vi "Image-correlation.vi"(6 "Image index":i32, 8 "error in":errorcluster, 9 "Correct. params. ref. in":refnum<data-value>, 10 "Buffer element in":T1 {"Temperature characteristics"."Stand. dev. temperature" format="%#.1f"; "Temperature characteristics"."Min. temperature" format="%#.0f"; "Temperature characteristics"."Max. temperature" format="%#.0f"; "Temperature characteristics"."Average temperature" format="%#.0f"}) -> (0 "error IO":errorcluster, 1 "Correct. params. ref.":refnum<data-value>, 2 "Buffer element":T1 {"Temperature characteristics"."Stand. dev. temperature" format="%#.1f"; "Temperature characteristics"."Min. temperature" format="%#.0f"; "Temperature characteristics"."Max. temperature" format="%#.0f"; "Temperature characteristics"."Average temperature" format="%#.0f"})   [LabVIEW 2013, in "CameraVision.lvlib" / "CV-Main.lvclass"]
uses:
  CV-Main.lvclass
  Correction/CV-Correction.lvclass
  Buffers/Storage-buffer.ctl
  <vilib>/vision/Image Controls.llb/IMAQ Image.ctl
  Temperature/Temperature-characteristics.ctl
  Analysis/Characteristics-cluster.ctl
  Correction/CV-Correction.lvclass/CV-Correction.ctl
  Correction/Read X-shift.vi
  Correction/Read Y-shift.vi
  Correction/Read Cross-correlation algorithm.vi
  Correction/Read Cross-correlation decimation.vi
  Correction/Write Image shift.vi
  Correction/Read Correlation algorithm.vi
  Correction/Read 2nd image correlation.vi
  Correction/Read 2nd image mirror axis.vi
  <vilib>/vision/NI_Vision_Development_Module.lvlib
  Temperature/CV-Temperature.lvclass
  Analysis/CV-Analysis.lvclass
  Buffers/CV-Buffers.lvclass
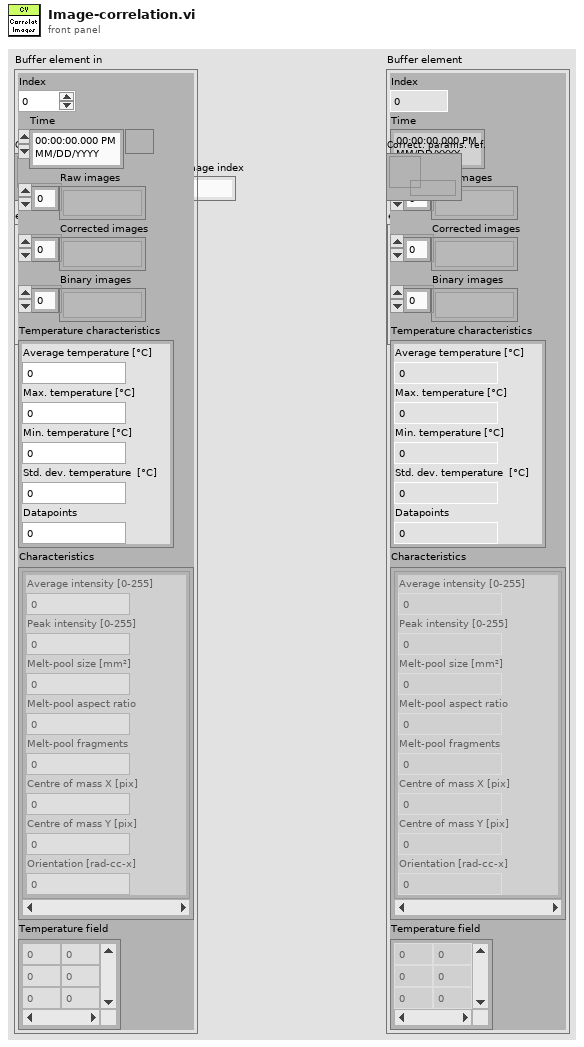
[diagram p1: front panel]
types:
  T1 = typedef "CameraVision.lvlib/CV-Buffers.lvclass/Storage-buffer.ctl" = cluster{"Index":i32, "Time":timestamp, "Raw images":T2[], "Corrected images":T2[], "Binary images":T2[], "Temperature characteristics":T3, "Characteristics":T4[], "Temperature field":dbl[][]}
  T2 = typedef "IMAQ Image.ctl" = refnum<image>
  T3 = typedef "CameraVision.lvlib/CV-Temperature.lvclass/Temperature-characteristics.ctl" = cluster{"Average temperature ":dbl, "Max. temperature":dbl, "Min. temperature":dbl, "Stand. dev. temperature":dbl, "Datapoints":dbl}
  T4 = typedef "CameraVision.lvlib/CV-Analysis.lvclass/Characteristics-cluster.ctl" = cluster{"Average intensity":dbl, "Peak intensity":dbl, "Melt-pool size":dbl, "Melt-pool aspect ratio":dbl, "Melt-pool fragments":dbl, "Centre of mass X":dbl, "Centre of mass Y":dbl, "Orientation":dbl}
  T5 = enum16{"Fixed shift", "Cross-correlation", "Cross-correlation (5steps)", "Melt-pool center"}
  T6 = cluster{"Accessors RO:X-shift":i32, "Accessors RO:Y-shift":i32}
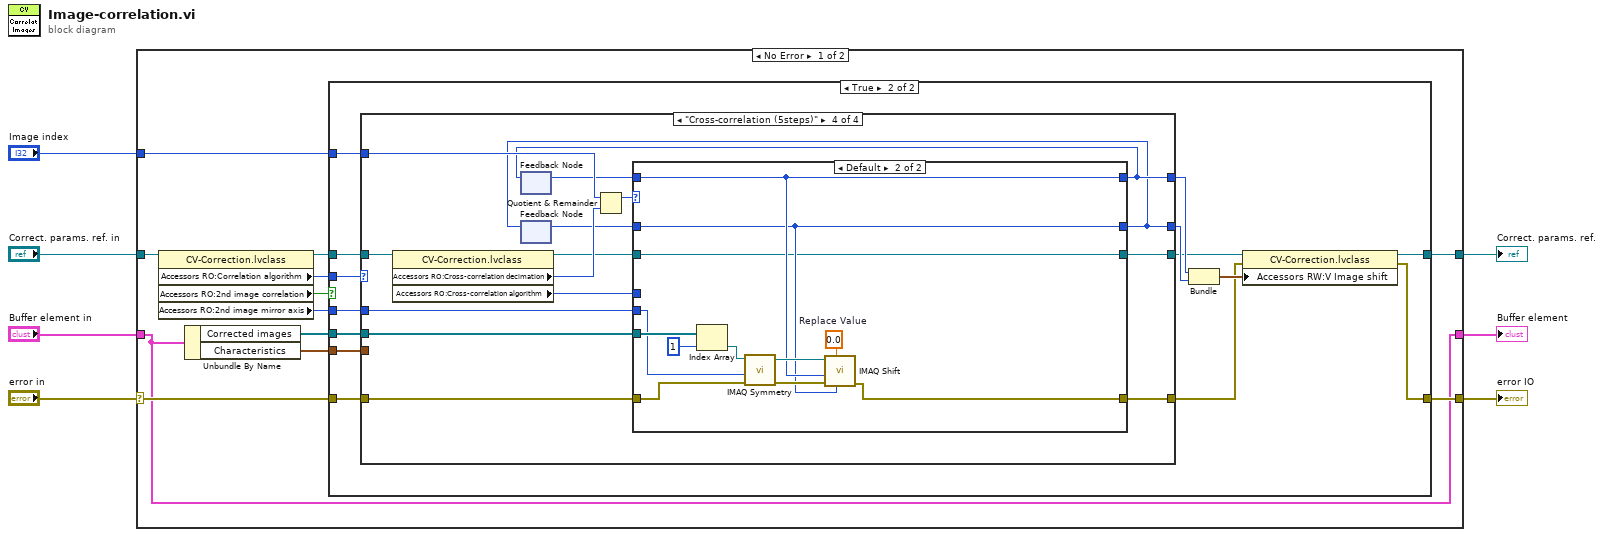
[diagram p0: block diagram]
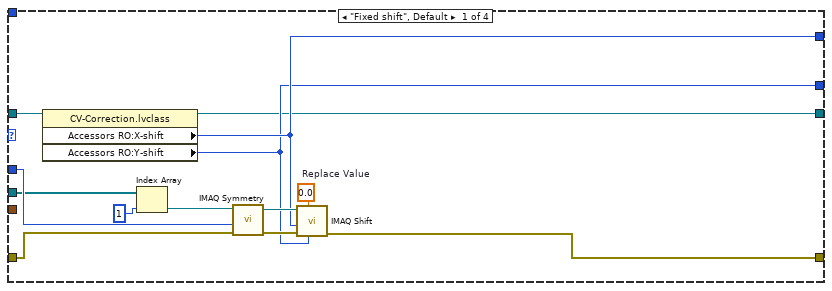
[diagram p3: hidden frame]
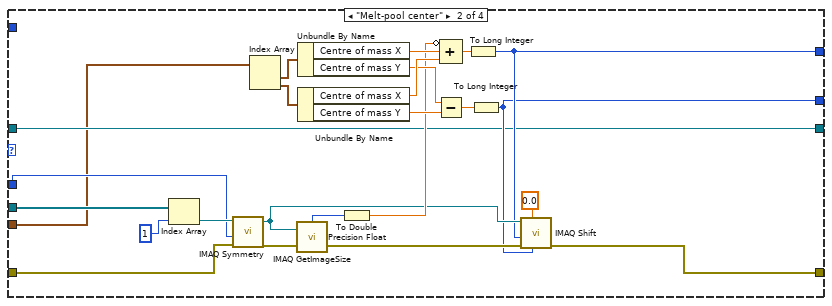
[diagram p4: hidden frame]
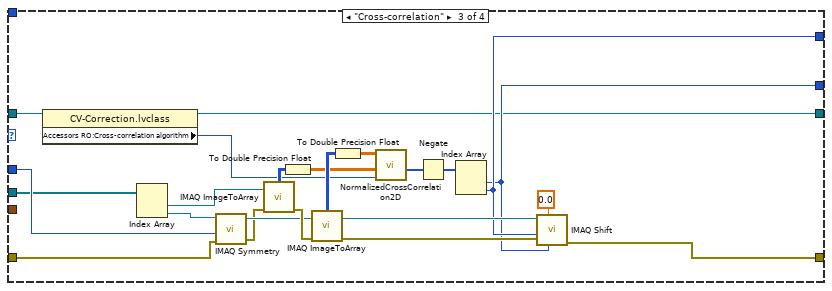
[diagram p5: hidden frame]
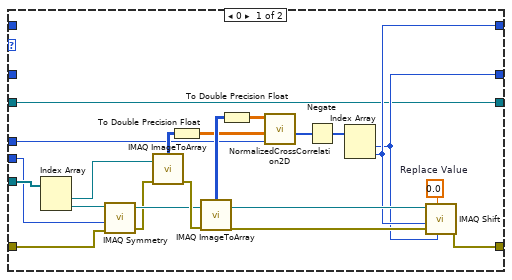
[diagram p6: hidden frame]
diagram:
  n1 = case shown="No Error" "error in" {
    selector: "error in" -> [w11 w145]
    tunnel: "Image index" -> [w19 _]
    tunnel: "Correct. params. ref. in" -> [w16 w144]
    tunnel: [w18 w145] -> w6
    tunnel: "Buffer element in" -> [w9 w143]
    tunnel: [w12 w144] -> w2
    tunnel: [w9 w143] -> w1
    frame No Error {
      n2 = property class="CV-Correction.lvclass"(reference=w16) -> (reference out=w17:refnum<data-value>, "Accessors RO:Correlation algorithm"=w15:T5, "Accessors RO:2nd image correlation"=w14:bool, "Accessors RO:2nd image mirror axis"=w13:u32)  [unwired: 1 in, 1 out]
      n3 = Unbundle By Name(w9) -> ("Corrected images"=w10:T2[], "Characteristics"=w8:T4[])
      n4 = case shown="True" w14 {
        tunnel: w19 -> [_ w35]
        tunnel: w15 -> [_ w34]
        tunnel: w17 -> [w21 w33]
        tunnel: [w20 w26] -> w18
        tunnel: w13 -> [_ w32]
        tunnel: [w21 w28] -> w12
        tunnel: w11 -> [w20 w24]
        tunnel: w10 -> [_ w23]
        tunnel: w8 -> [_ w22]
        frame False {
        }
        frame True {
          n5 = case shown="\"Cross-correlation (5steps)\"" w34 {
            tunnel: [w39 w53 w76 w107] -> w25
            tunnel: w33 -> [w42 w52 w81 w106]
            tunnel: w35 -> [_ _ _ w109]
            tunnel: w32 -> [w43 w57 w79 w102]
            tunnel: [w41 w55 w78 w101] -> w31
            tunnel: [w40 w54 w77 w99] -> w30
            tunnel: [w38 w52 w75 w97] -> w29
            tunnel: w24 -> [w36 w51 w74 w96]
            tunnel: w23 -> [w37 w50 w73 w95]
            tunnel: w22 -> [_ w49 _ _]
            frame "Fixed shift", Default {
              w48 = sgl 0.0  # Replace Value
              n6 = property class="CV-Correction.lvclass"(reference=w42) -> (reference out=w38:refnum<data-value>, "Accessors RO:X-shift"=w41:i32, "Accessors RO:Y-shift"=w40:i32)  [unwired: 1 in, 1 out]
              n7 = Index Array(array=w37, index=1) -> (element=w47:T2)
              n8 = call "IMAQ Symmetry"("error in (no error)"=w36, "Type of Symmetry"=w43, "Image Src"=w47) -> ("error out"=w44:errorcluster, "Image Dst Out"=w45:T2)  [unwired: 2 in]
              n9 = call "IMAQ Shift"("YOffset"=w40, "Replace Value"=w48, "error in (no error)"=w44, "XOffset"=w41, "Image Src"=w45) -> ("error out"=w39:errorcluster)  [unwired: 5 in, 1 out]
            }
            frame "Melt-pool center" {
              n10 = Index Array(array=w50, index=1) -> (element=w63:T2)
              n11 = call "IMAQ Symmetry"("error in (no error)"=w51, "Type of Symmetry"=w57, "Image Src"=w63) -> ("error out"=w61:errorcluster, "Image Dst Out"=w56:T2)  [unwired: 2 in]
              n12 = Index Array(array=w49) -> (element #1=w72:T4, element #2=w71:T4)  [unwired: 2 in]
              n13 = call "IMAQ GetImageSize"("Image"=w56, "error in (no error)"=w61) -> ("X Resolution"=w59:i32, "error out"=w60:errorcluster)  [unwired: 2 in, 1 out]
              n14 = Unbundle By Name(w72) -> ("Centre of mass X"=w70:dbl, "Centre of mass Y"=w67:dbl)
              n15 = Unbundle By Name(w71) -> ("Centre of mass X"=w69:dbl, "Centre of mass Y"=w68:dbl)
              n16 = To Double Precision Float(number=w59) -> (double precision float=w58:dbl)
              n17 = Subtract(x=w67, y=w68) -> (x-y=w65:dbl)
              n18 = Compound Arithmetic op=ADD(invert w58, w70, w69) -> (w66:dbl)
              n19 = To Long Integer(number=w66) -> (32bit integer=w55:i32)
              n20 = To Long Integer(number=w65) -> (32bit integer=w54:i32)
              n21 = call "IMAQ Shift"("YOffset"=w54, "Replace Value"=sgl 0.0, "error in (no error)"=w60, "XOffset"=w55, "Image Src"=w56) -> ("error out"=w53:errorcluster)  [unwired: 5 in, 1 out]
            }
            frame "Cross-correlation" {
              n22 = property class="CV-Correction.lvclass"(reference=w81) -> (reference out=w75:refnum<data-value>, "Accessors RO:Cross-correlation algorithm"=w80:enum32{"direct", "frequency domain"})  [unwired: 1 in, 1 out]
              n23 = Index Array(array=w73) -> (element #1=w82:T2, element #2=w86:T2)  [unwired: 2 in]
              n24 = call "IMAQ Symmetry"("error in (no error)"=w74, "Type of Symmetry"=w79, "Image Src"=w86) -> ("error out"=w84:errorcluster, "Image Dst Out"=w85:T2)  [unwired: 2 in]
              n25 = call "IMAQ ImageToArray"("error in (no error)"=w84, "Image"=w82) -> ("error out"=w91:errorcluster, "Image Pixels (U8)"=w93:u8[][])  [unwired: 2 in, 3 out]
              n26 = To Double Precision Float(number=w93) -> (double precision float=w89:dbl[][])
              n27 = call "IMAQ ImageToArray"("error in (no error)"=w91, "Image"=w85) -> ("error out"=w90:errorcluster, "Image Pixels (U8)"=w94:u8[][])  [unwired: 2 in, 3 out]
              n28 = To Double Precision Float(number=w94) -> (double precision float=w92:dbl[][])
              n29 = call "NormalizedCrossCorrelation2D.vi"("Correlation Domain"=w80, "Template"=w89, "Array"=w92) -> ("Maximum Indices"=w88:i32[])  [unwired: 6 in, 2 out]
              n30 = Negate(x=w88) -> (-x=w87:i32[])
              n31 = Index Array(array=w87) -> (element #1=w77:i32, element #2=w78:i32)  [unwired: 2 in]
              n32 = call "IMAQ Shift"("YOffset"=w77, "Replace Value"=sgl 0.0, "error in (no error)"=w90, "XOffset"=w78, "Image Src"=w85) -> ("error out"=w76:errorcluster)  [unwired: 5 in, 1 out]
            }
            frame "Cross-correlation (5steps)" {
              n33 = property class="CV-Correction.lvclass"(reference=w106) -> (reference out=w103:refnum<data-value>, "Accessors RO:Cross-correlation decimation"=w105:i32, "Accessors RO:Cross-correlation algorithm"=w104:enum32{"direct", "frequency domain"})  [unwired: 1 in, 1 out]
              n34 = feedback #1() -> (w100:i32)  [unwired: 1 in]
              n35 = feedback #2() -> (w98:i32)  [unwired: 1 in]
              n36 = Quotient & Remainder(x=w109, y=w105) -> (x-y*floor(x/y)=w108:i32)  [unwired: 1 out]
              n37 = case shown="Default" w108 {
                tunnel: [w113 w133] -> w107
                tunnel: w95 -> [w117 w140]
                tunnel: w104 -> [w116 _]
                tunnel: w103 -> [w110 w131]
                tunnel: w96 -> [w114 w132]
                tunnel: w102 -> [w115 w136]
                tunnel: [w112 w135] -> w101
                tunnel: [w111 w134] -> w99
                tunnel: w100 -> [_ w135]
                tunnel: w98 -> [_ w134]
                tunnel: [w110 w131] -> w97
                frame 0 {
                  w119 = sgl 0.0  # Replace Value
                  n38 = Index Array(array=w117) -> (element #1=w118:T2, element #2=w122:T2)  [unwired: 2 in]
                  n39 = call "IMAQ Symmetry"("error in (no error)"=w114, "Type of Symmetry"=w115, "Image Src"=w122) -> ("error out"=w120:errorcluster, "Image Dst Out"=w121:T2)  [unwired: 2 in]
                  n40 = call "IMAQ ImageToArray"("error in (no error)"=w120, "Image"=w118) -> ("error out"=w127:errorcluster, "Image Pixels (U8)"=w129:u8[][])  [unwired: 2 in, 3 out]
                  n41 = To Double Precision Float(number=w129) -> (double precision float=w125:dbl[][])
                  n42 = call "IMAQ ImageToArray"("error in (no error)"=w127, "Image"=w121) -> ("error out"=w126:errorcluster, "Image Pixels (U8)"=w130:u8[][])  [unwired: 2 in, 3 out]
                  n43 = To Double Precision Float(number=w130) -> (double precision float=w128:dbl[][])
                  n44 = call "NormalizedCrossCorrelation2D.vi"("Correlation Domain"=w116, "Template"=w125, "Array"=w128) -> ("Maximum Indices"=w124:i32[])  [unwired: 6 in, 2 out]
                  n45 = Negate(x=w124) -> (-x=w123:i32[])
                  n46 = Index Array(array=w123) -> (element #1=w111:i32, element #2=w112:i32)  [unwired: 2 in]
                  n47 = call "IMAQ Shift"("YOffset"=w111, "Replace Value"=w119, "error in (no error)"=w126, "XOffset"=w112, "Image Src"=w121) -> ("error out"=w113:errorcluster)  [unwired: 5 in, 1 out]
                }
                frame Default {
                  w141 = sgl 0.0  # Replace Value
                  n48 = Index Array(array=w140, index=1) -> (element=w138:T2)
                  n49 = call "IMAQ Symmetry"("error in (no error)"=w132, "Type of Symmetry"=w136, "Image Src"=w138) -> ("error out"=w137:errorcluster, "Image Dst Out"=w142:T2)  [unwired: 2 in]
                  n50 = call "IMAQ Shift"("YOffset"=w134, "Replace Value"=w141, "error in (no error)"=w137, "XOffset"=w135, "Image Src"=w142) -> ("error out"=w133:errorcluster)  [unwired: 5 in, 1 out]
                }
              }
              n51 = feedback-in #1(w101) -> ()
              n52 = feedback-in #2(w99) -> ()
            }
          }
          n53 = Bundle("Accessors RO:X-shift"=w31, "Accessors RO:Y-shift"=w30) -> (w27:T6)  [unwired: 1 in]
          n54 = property class="CV-Correction.lvclass"(reference=w29, error in=w25, "Accessors RW:V Image shift"=w27) -> (reference out=w28:refnum<data-value>, error out=w26:errorcluster)
        }
      }
    }
    frame Error {
    }
  }
  "error IO" <- w6
  "Buffer element" <- w1
  "Correct. params. ref." <- w2
